vi "Tran to CRC.vi"(5 "CheckSum？":bool, 7 "Count":bool, 8 "MessageFrame":refnum<k21>="ESP_1\nLRA110", 9 "校验算法名称":string="Anti_Add", 11 "CAN_commd":dbl[](array[numeric])=[50.0, 1.0, 11.0, 0.0, 0.0, 0.0, 0.0, 0.0, 0.0] caption="data") -> (1 "Output CAN Command":u8[](array[numeric]) format="%x", 2 "校验值":u64 format="%.0x", 3 "SignalsArryOut":dbl[](array[numeric]))   [LabVIEW 2020]
panel:
  out "CAN_Command_U8":u8[](array[numeric]) format="%.0x"
  # "speedStatus"
  # "counter"
  # "speed"
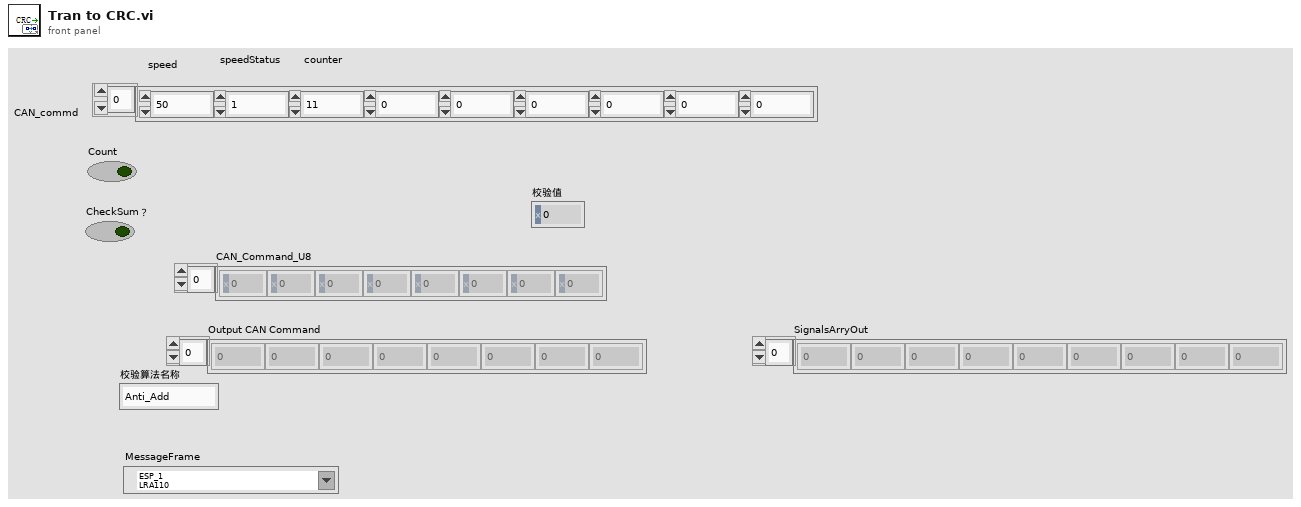
[diagram p1: front panel]
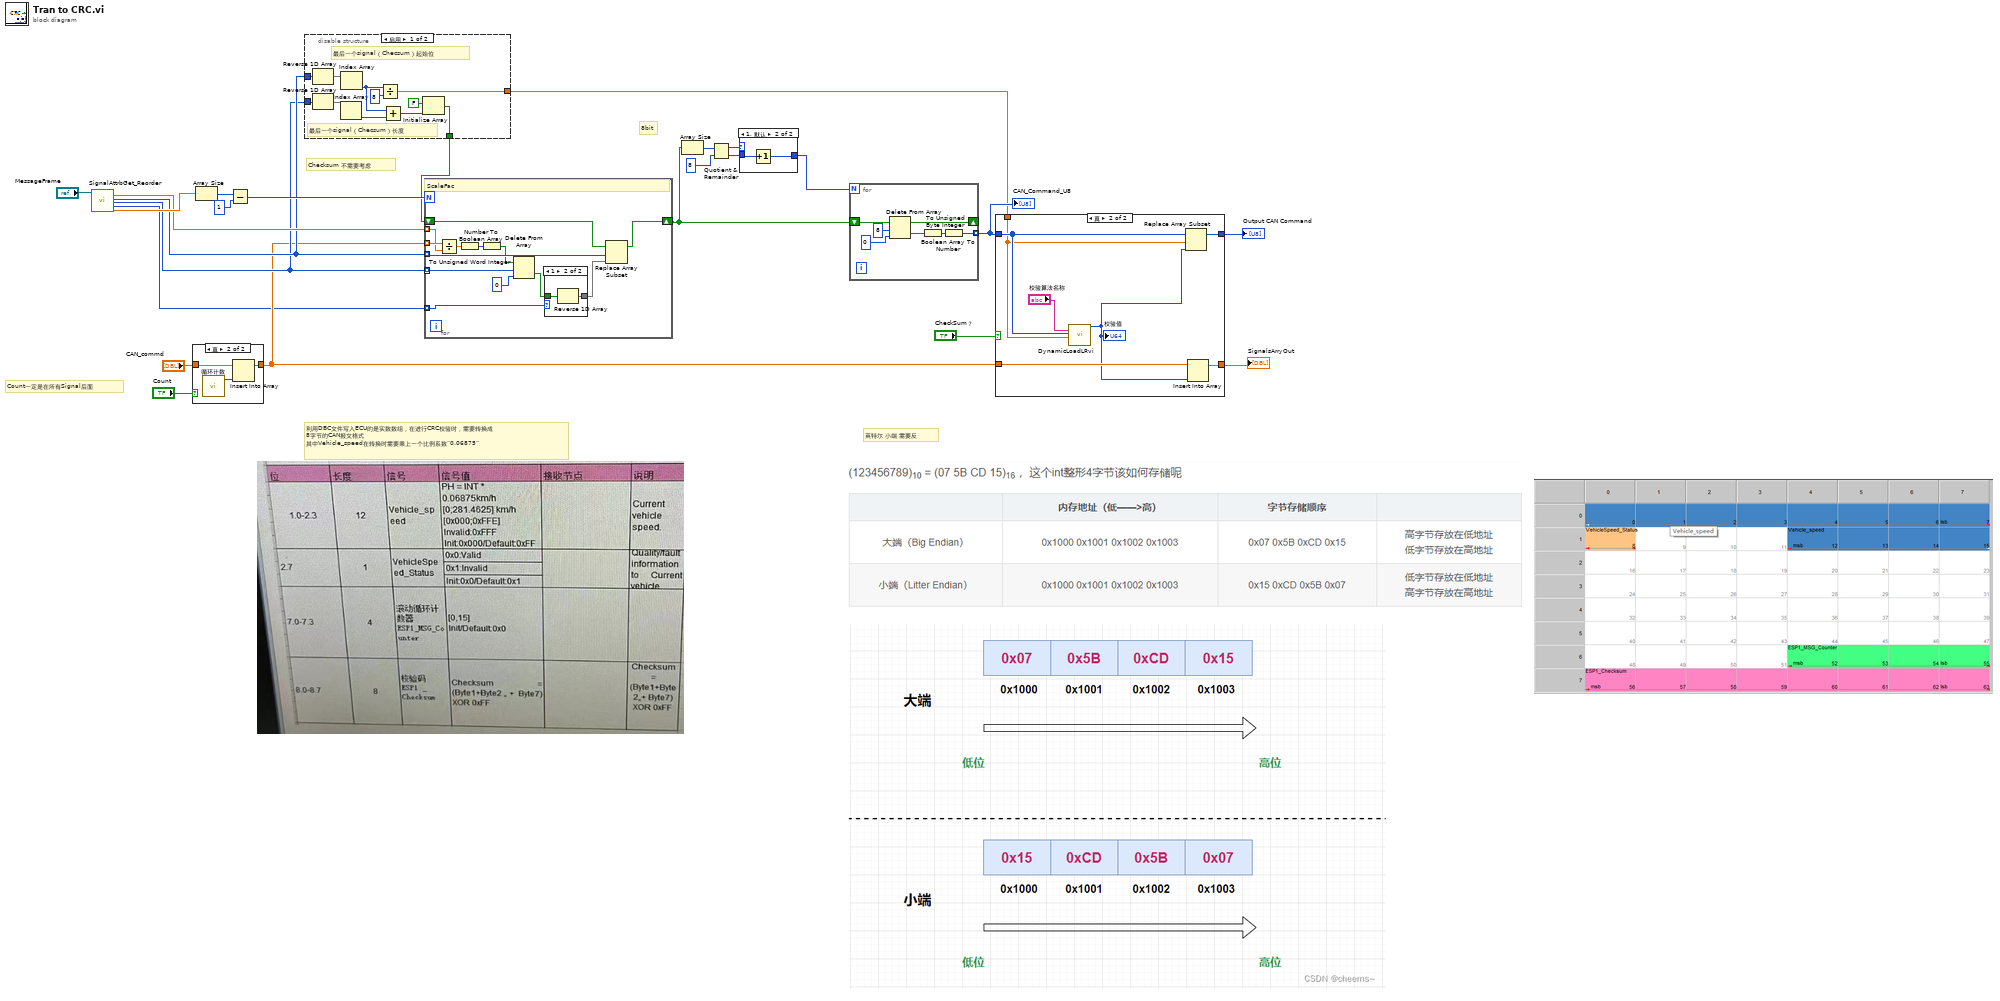
[diagram p0: block diagram]
diagram:
  # "Count一定是在所有Signal后面"
  # "8bit"
  # "Checksum 不需要考虑"
  # "英特尔 小端 需要反"
  # "利用DBC文件写入ECU的是实数数组，在进行CRC校验时，需要转换成\n8字节的CAN报文格式\n其中Vehicle_speed在转换时需要乘上一个比例系数“0.06875”"
  n1 = call "SignalAttrbGet_Reorder.vi"("MessageFrame"="MessageFrame") -> ("ScaleFac"=w19:dbl[], "StartBitArry"=w17:u32[], "Length"=w16:u32[], "DataType"=w7:u32[], "DefaultValue"=w22:dbl[])  [unwired: 12 in, 2 out]
  n2 = case shown="真" "Count" {
    tunnel: "CAN_commd" -> [w25 w28]
    tunnel: [w25 w26] -> w9
    frame False {
    }
    frame True {
      n3 = call "循环计数.vi"() -> ("循环计数"=w27:u8)  [unwired: 11 in]
      n4 = Insert Into Array(array=w28, new element=w27) -> (w26:dbl[])  [unwired: 1 in]
    }
  }
  n5 = Array Size(array=w22) -> (size(s)=w21:i32)
  n6 = Subtract(x=w21, y=1 ("x")) -> (x-y=w20:i32)
  n7 = disable-structure shown="启用" {
    disable-tunnel: w17 -> [w39 _]
    disable-tunnel: w16 -> [w38 _]
    disable-tunnel: [w34 _] -> w14
    disable-tunnel: [w29 _] -> w13
    frame Enabled {
      # "最后一个signal（Checsum）长度"
      # "最后一个signal（Checsum）起始位"
      n8 = Reverse 1D Array(array=w39) -> (reversed array=w37:u32[])
      n9 = Reverse 1D Array(array=w38) -> (reversed array=w36:u32[])
      n10 = Index Array(array=w36) -> (element=w32:u32)  [unwired: 1 in]
      n11 = Index Array(array=w37) -> (element=w33:u32)  [unwired: 1 in]
      n12 = Divide(x=w33, y=8) -> (x/y=w34:dbl)
      n13 = Add(x=w33, y=w32) -> (x+y=w30:u32)
      n14 = Initialize Array(FALSE, w30) -> (w29:bool[])
    }
    frame Disabled {
    }
  }
  n15 = for {
    N: w20 -> [_]
    tunnel: w9 -> [w52] mode=indexing
    tunnel: w19 -> [w51] mode=indexing
    tunnel: w17 -> [w46] mode=indexing
    shift-right: [w47] -> w6
    shift-left: w13 -> [w48]
    tunnel: w16 -> [w43] mode=indexing
    tunnel: w7 -> [w42] mode=indexing
    # "ScaleFac"
    n16 = Divide(x=w52, y=w51) -> (x/y=w50:dbl)
    n17 = To Unsigned Word Integer(number=w50) -> (unsigned 16bit integer=w49:u16)
    n18 = Number To Boolean Array(number=w49) -> (Boolean array=w44:bool[])
    n19 = Delete From Array(array=w44, length=w43, index=0) -> (deleted portion=w41:bool[])  [unwired: 1 out]
    n20 = case shown="1" w42 {
      tunnel: w41 -> [w53 w55]
      tunnel: [w53 w54] -> w40
      frame 0, Default {
        # "小端\nIntel"
      }
      frame 1 {
        n21 = Reverse 1D Array(array=w55) -> (reversed array=w54:bool[])
      }
    }
    n22 = Replace Array Subset(array=w48, new element=w40, index=w46) -> (w47:bool[])
  }
  n23 = Array Size(array=w6) -> (size(s)=w5:i32)
  n24 = Quotient & Remainder(x=w5, y=8) -> (x-y*floor(x/y)=w3:i32, floor(x/y)=w2:i32)
  n25 = case shown="1, 默认" w3 {
    tunnel: w2 -> [w56 w58]
    tunnel: [w56 w57] -> w1
    frame 0 {
    }
    frame 1, Default {
      n26 = Increment(x=w58) -> (x+1=w57:i32)
    }
  }
  n27 = for {
    N: w1 -> [_]
    shift-right: [w61] -> _
    shift-left: w6 -> [w65]
    tunnel: [w59] -> w15 mode=indexing
    n28 = Delete From Array(array=w65, length=8, index=0) -> (deleted portion=w62:bool[], array with subset deleted=w61:bool[])
    n29 = Boolean Array To Number(Boolean array=w62) -> (number=w60:u16)
    n30 = To Unsigned Byte Integer(number=w60) -> (unsigned 8bit integer=w59:u8)
  }
  "CAN_Command_U8" <- w15
  n31 = case shown="真" "CheckSum？" {
    tunnel: [w66 w74] -> w24
    tunnel: w15 -> [w66 w70]
    tunnel: w14 -> [_ w69]
    tunnel: w9 -> [w67 w73]
    tunnel: [w67 w72] -> w8
    frame False {
    }
    frame True {
      n32 = call "DynamicLoadLRvi.vi"("校验算法名称"="校验算法名称", "校验数据"=w70, "校验长度"=w69) -> ("校验值"=w68:u64)  [unwired: 16 in]
      "校验值" <- w68
      n33 = Replace Array Subset(array=w70, new element=w68, index=w69) -> (w74:u8[])
      n34 = Insert Into Array(array=w73, new element=w68) -> (w72:dbl[])  [unwired: 1 in]
    }
  }
  "Output CAN Command" <- w24
  "SignalsArryOut" <- w8
